vi "F_array_to_8bit_BMP_file.vi"(8 "error in (no error)":errorcluster, 10 "2D array in":u8[][](array[numeric]), 11 "path to save BMP file":path) -> (0 "error out":errorcluster)   [LabVIEW 2016]
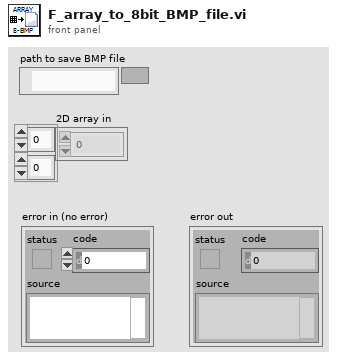
[diagram p1: front panel]
types:
  T1 = typedef "Image Type" = u32
  T2 = typedef "IMAQ Image.ctl" = refnum<image>
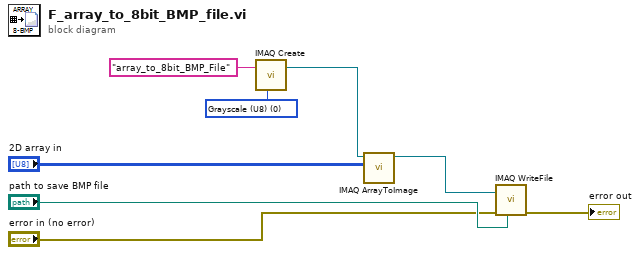
[diagram p0: block diagram]
diagram:
  w8 = T1 0 items=["Grayscale (U8)", "Grayscale (I16)", "Grayscale (SGL)", "Complex (CSG)", "RGB (U32)", "HSL (U32)", "RGB (U64)", "Grayscale (U16)"] ("Image Type")
  n1 = call "IMAQ Create"("Image Name"="array_to_8bit_BMP_File", "Image Type"=w8) -> ("New Image"=w5:T2)  [unwired: 3 in, 1 out]
  n2 = call "IMAQ ArrayToImage"("Image Pixels (U8)"="2D array in", "Image"=w5) -> ("Image Out"=w4:T2)  [unwired: 8 in, 1 out]
  n3 = call "IMAQ WriteFile"("error in (no error)"="error in (no error)", "File Path"="path to save BMP file", "Image"=w4) -> ("error out"=→"error out":errorcluster)  [unwired: 5 in]
